vi "Search ADALM2000.vi"() -> (3 "Array":string[](array[string]))   [LabVIEW 2015]
uses:
  libm2k_lv.dll
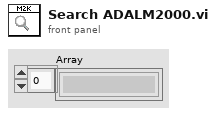
[diagram p1: front panel]
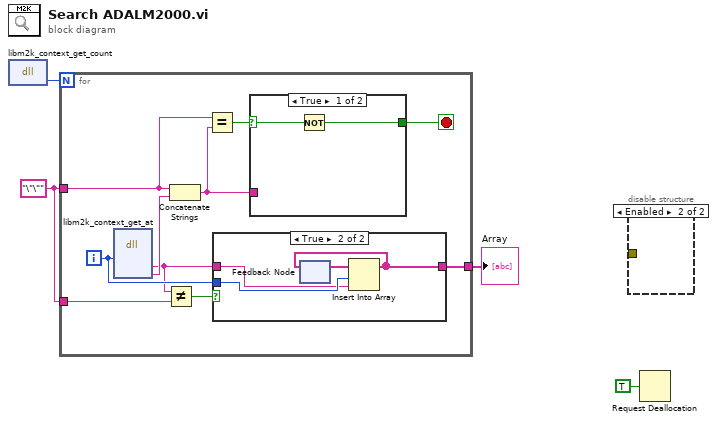
[diagram p0: block diagram]
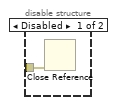
[diagram p2: hidden frame]
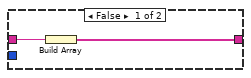
[diagram p3: hidden frame]
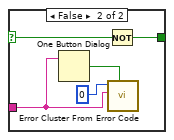
[diagram p4: hidden frame]
diagram:
  w3 = "\"\""
  n1 = dll-call lib="libm2k_lv.*" fn="libm2k_context_get_count"() -> ("return type"=w4:i64)  [unwired: 3 in, 2 out]
  n2 = for {
    N: w4 -> [_]
    tunnel: w3 -> [w13]
    tunnel: w3 -> [w9]
    tunnel: [w5] -> w2
    i -> [w7]
    stop <- w10 stop-if-true
    n3 = dll-call lib="libm2k_lv.*" fn="libm2k_context_get_at"("uri_idx"=w7) -> ("uri"=w6:string, "err"=w14:string)  [unwired: 7 in, 2 out]
    n4 = Not Equal?(x=w6, y=w9) -> (x != y?=w8:bool)
    n5 = Concatenate Strings(w13, w14) -> (w12:string)
    n6 = Equal?(x=w13, y=w12) -> (x = y?=w11:bool)
    n7 = case shown="True" w8 {
      tunnel: w7 -> [_ w20]
      tunnel: w6 -> [w15 w19]
      tunnel: [w16 w17] -> w5
      frame False {
        n8 = Build Array(w15) -> (w16:string[])
      }
      frame True {
        n9 = feedback #1() -> (w18:string[])  [unwired: 1 in]
        n10 = Insert Into Array(array=w18, index=w20, new element=w19) -> (w17:string[])
        n11 = feedback-in #1(w17) -> ()
      }
    }
    n12 = case shown="True" w11 {
      selector: w11 -> [w22 w24]
      tunnel: w12 -> [_ w25]
      tunnel: [w21 w23] -> w10
      frame True {
        n13 = Not(x=w22) -> (.not. x?=w21:bool)
      }
      frame False {
        n14 = One Button Dialog(message=w25) -> (true=w27:bool)  [unwired: 1 in]
        n15 = Not(x=w24) -> (.not. x?=w23:bool)
        n16 = call <vilib>:"Error Cluster From Error Code.vi"("show call chain? (False)"=w27, "error message (\"\")"=w25, "error code (0)"=0) -> ()  [unwired: 6 in, 1 out]
      }
    }
  }
  "Array" <- w2
  n17 = disable-structure shown="Enabled" {
    disable-tunnel: _ -> [w28 _]
    frame Disabled {
      n18 = Close Reference(error in (no error)=w28) -> ()  [unwired: 1 in, 1 out]
    }
    frame Enabled {
    }
  }
  n19 = Request Deallocation(TRUE ("flag")) -> ()
